vi "oa_Check Reset (1 Channel).vi"(7 "reset?":bool=TRUE, 8 "error in (no error)":errorcluster, 10 "empty signal?":bool, 11 "resampled signal":cluster{"r0":dbl, "dr":dbl, "Y":dbl[]} {"r0" format="%.2p"; "dr" format="%.2p"; "Y" format="%.2f"}) -> (0 "error out":errorcluster, 2 "reset out?":bool, 3 "resampled signal dup":cluster{"r0":dbl, "dr":dbl, "Y":dbl[]} {"r0" format="%.2p"; "dr" format="%.2p"; "Y" format="%.2f"})   [LabVIEW 2017, in "SoundVib_Resampling.lvlib"]
uses:
  <vilib>/addons/Sound and Vibration/Order Analysis/Resample Order Tracking/SoundVib_Resampling.lvlib
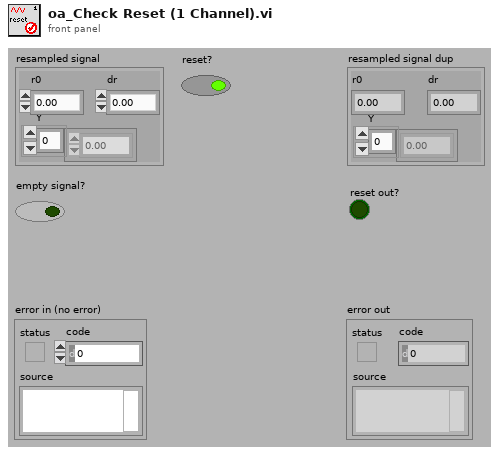
[diagram p1: front panel]
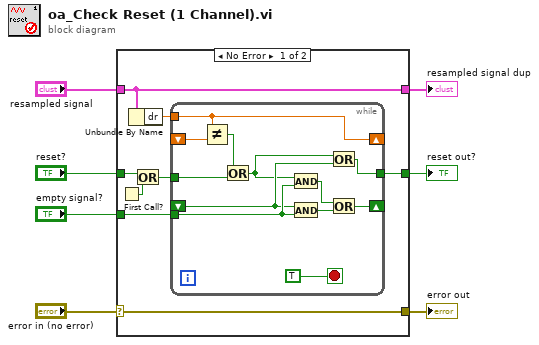
[diagram p0: block diagram]
diagram:
  n1 = case shown="No Error" "error in (no error)" {
    selector: "error in (no error)" -> [w15 w30]
    tunnel: [w15 w30] -> w6
    tunnel: "reset?" -> [w12 w29]
    tunnel: "empty signal?" -> [w14 _]
    tunnel: "resampled signal" -> [w9 w28]
    tunnel: [w9 w28] -> w2
    tunnel: [w13 w29] -> w1
    frame No Error {
      n2 = First Call?() -> (First Call?: T/F=w11:bool)
      n3 = Unbundle By Name(w9) -> ("dr"=w8:dbl)
      n4 = Or(x=w12, y=w11) -> (x .or. y?=w10:bool)
      n5 = while {
        tunnel: w10 -> [w17]
        tunnel: w14 -> [w22]
        shift-right: [w24] -> _
        shift-left: _ -> [w21]
        tunnel: [w23] -> w13
        shift-right: [w19] -> _
        shift-left: _ -> [w20]
        tunnel: w8 -> [w19]
        stop <- TRUE stop-if-true
        n6 = Not Equal?(x=w19, y=w20) -> (x != y?=w18:bool)
        n7 = Or(x=w18, y=w17) -> (x .or. y?=w16:bool)
        n8 = And(x=w16, y=w22) -> (x .and. y?=w26:bool)
        n9 = And(x=w21, y=w22) -> (x .and. y?=w25:bool)
        n10 = Or(x=w16, y=w21) -> (x .or. y?=w23:bool)
        n11 = Or(x=w26, y=w25) -> (x .or. y?=w24:bool)
      }
    }
    frame Error {
    }
  }
  "resampled signal dup" <- w2
  "error out" <- w6
  "reset out?" <- w1
